vi "20170411-lecture3-local variable.vi"() -> ()   [LabVIEW 2014]
uses:
  20170411-lecture3-global variable.vi
panel:
  out "Chart 2":dbl(graph)
  in  "stop":bool
  out "Chart 1":dbl(graph)
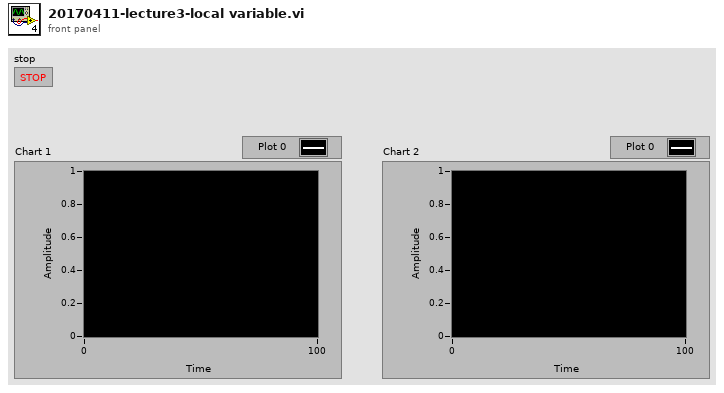
[diagram p1: front panel]
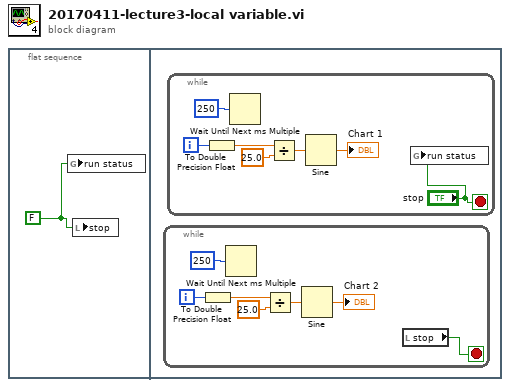
[diagram p0: block diagram]
diagram:
  n1 = flat-sequence {
    frame #0 {
      w1 = FALSE
      n2 = global write "20170411-lecture3-global variable.vi" "run status"(w1) -> ()
      n3 = local write "stop"(w1) -> ()
    }
    frame #1 {
      n4 = while {
        i -> [w3]
        stop <- w2 stop-if-true
        n5 = To Double Precision Float(number=w3) -> (double precision float=w4:dbl)
        n6 = Wait Until Next ms Multiple(millisecond multiple=u32 250) -> ()  [unwired: 1 out]
        n7 = Divide(x=w4, y=25.0) -> (x/y=w8:dbl)
        n8 = Sine(x=w8) -> (sin(x)=→"Chart 2":dbl)
        n9 = local read "stop"() -> (w2:bool)
      }
      n10 = while {
        i -> [w10]
        stop <- "stop" stop-if-true
        n11 = To Double Precision Float(number=w10) -> (double precision float=w11:dbl)
        n12 = Wait Until Next ms Multiple(millisecond multiple=u32 250) -> ()  [unwired: 1 out]
        n13 = Divide(x=w11, y=25.0) -> (x/y=w15:dbl)
        n14 = Sine(x=w15) -> (sin(x)=→"Chart 1":dbl)
        n15 = global write "20170411-lecture3-global variable.vi" "run status"("stop") -> ()
      }
    }
  }
